vi "DP-Init Data File.vi"(2 "Path":path, 5 "Parameters":T2, 11 "error in (no error)":errorcluster) -> (15 "error out":errorcluster)   [LabVIEW 2020]
uses:
  Typedefs/DP-Parameters.ctl
  Typedefs/DP-Stimulus Params.ctl
  Typedefs/DP-Response Params.ctl
  Typedefs/DP-Data Header.ctl
  epl-vi-lib/Utility VIs/File IO VIs/Configuration File Wrapper VIs/Config-Read Key (string).vi
  CFTS VIs/CFTS-Globals.vi
panel:
  in  "DPOAE I-O":T1
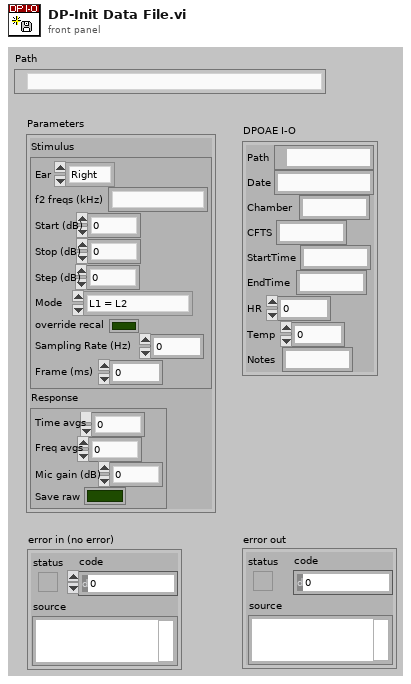
[diagram p1: front panel]
types:
  T1 = typedef "DP-Data Header.ctl" = cluster{"Path":path, "Date":string, "Chamber":string, "CFTS":string, "StartTime":string, "EndTime":string, "HR":dbl, "Temp":dbl, "Notes":string}
  T2 = typedef "DP-Parameters.ctl" = cluster{"Stimulus":T3, "Response":T4}
  T3 = typedef "DP-Stimulus Params.ctl" = cluster{"Ear":enum16{"Right", "Left"}, "f2 freqs (kHz)":string, "Start (dB)":dbl, "Stop (dB)":dbl, "Step (dB)":dbl, "Mode":enum16{"L1 = L2", "L1 = L2 + 10 dB"}, "override recal":bool, "Sampling Rate (Hz)":dbl, "Frame (ms)":dbl}
  T4 = typedef "DP-Response Params.ctl" = cluster{"Time avgs":i32, "Freq avgs":i32, "Mic gain (dB)":dbl, "Save raw":bool}
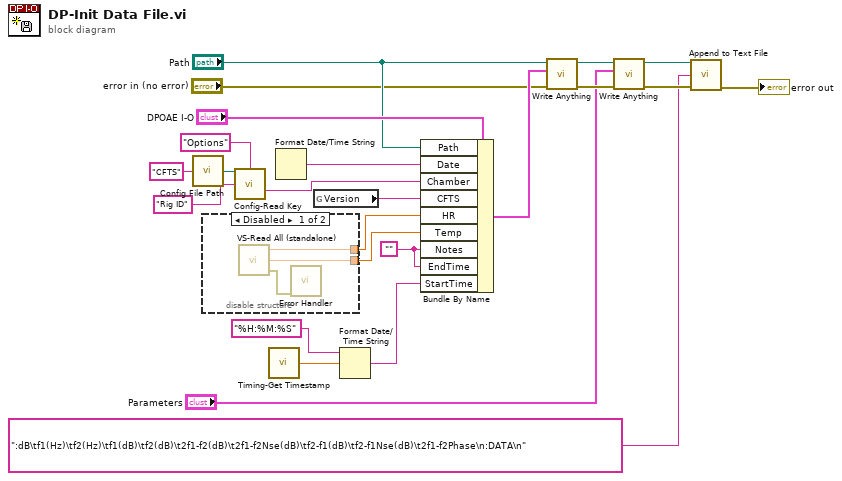
[diagram p0: block diagram]
diagram:
  w4 = ""
  n1 = call "Config File Path.vi"("AppName"="CFTS") -> ("Default config file name"=w22:path)
  n2 = disable-structure shown="Disabled" {
    disable-tunnel: [w27 _] -> w16
    disable-tunnel: [w26 _] -> w15
    frame Disabled {
      n3 = call "VS-Read All (standalone).vi"() -> ("error out"=w25:errorcluster, "Heart Rate (bpm)"=w26:dbl, "Temperature (C)"=w27:dbl)  [unwired: 3 in]
      n4 = call "Error Handler.vi"("error in (no error)"=w25) -> ()  [unwired: 12 in, 3 out]
    }
    frame Enabled {
    }
  }
  n5 = call-poly "Config-Read Key.vi"("configuration file path"=w22, "section"="Options", "key"="Rig ID" ("string")) -> ("value"=w18:string)  [unwired: 9 in, 3 out]
  n6 = call "Timing-Get Timestamp.vi"() -> ("double precision float"=w3:dbl)  [unwired: 14 in, 1 out]
  n7 = Format Date/Time String() -> (date/time string=w19:string)  [unwired: 3 in]
  n8 = global read "CFTS-Globals.vi" "Version"() -> (w17:string)
  n9 = Format Date/Time String(time format string (%c)="%H:%M:%S", seconds (now)=w3) -> (date/time string=w1:string)  [unwired: 1 in]
  n10 = Bundle By Name(cluster="DPOAE I-O", "Path"="Path", "Date"=w19, "Chamber"=w18, "CFTS"=w17, "HR"=w16, "Temp"=w15, "Notes"=w4, "EndTime"=w4, "StartTime"=w1) -> (w11:T1)
  n11 = call "Write Anything.vi"("Error In"="error in (no error)", "Anything"=w11, "Path (dialog)"="Path") -> ("Error Out"=w13:errorcluster, "Path out"=w14:path)  [unwired: 7 in]
  n12 = call "Write Anything.vi"("Error In"=w13, "Anything"="Parameters", "Path (dialog)"=w14) -> ("Error Out"=w7:errorcluster, "Path out"=w8:path)  [unwired: 7 in]
  n13 = call "Append to Text File.vi"("file path"=w8, "text"=":dB\tf1(Hz)\tf2(Hz)\tf1(dB)\tf2(dB)\t2f1-f2(dB)\t2f1-f2Nse(dB)\tf2-f1(dB)\tf2-f1Nse(dB)\t2f1-f2Phase\n:DATA\n", "error in (no error)"=w7) -> ("error out"=→"error out":errorcluster)  [unwired: 11 in, 1 out]
